vi "压力测试.vi"(15 "stop":bool) -> ()   [LabVIEW 2010]
uses:
  Instance           1 16Saved   压力测试 .vi
  Instance           2 16Saved   压力测试 .vi
  <vilib>/Analysis/NI_AALBase.lvlib
panel:
  in  "量  程(MPa)":dbl=5.0
  in  "零点输出(mV)":dbl=0.183
  in  "输出灵敏度（mV/V）":dbl=1.399
  out "当前压力值(MPa)":dbl(knob)=1.5270779105911612 scale=0.0..5.0
  out "压力 (Mpa)":dbl(graph)=1.31 caption="压力曲线 (Mpa)"
  # "压力测量实验"
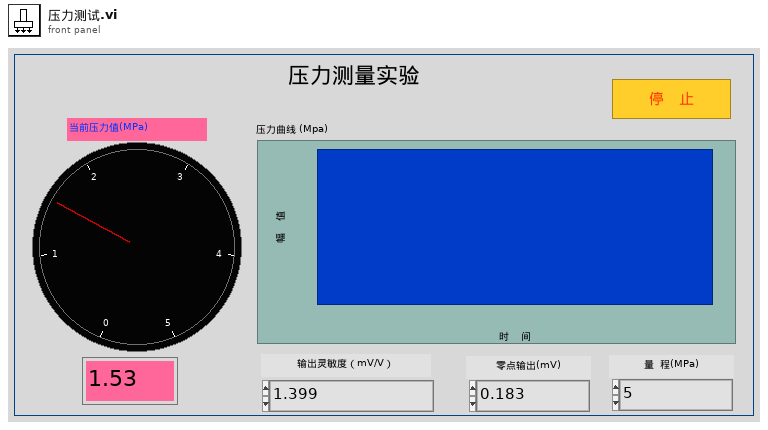
[diagram p1: front panel]
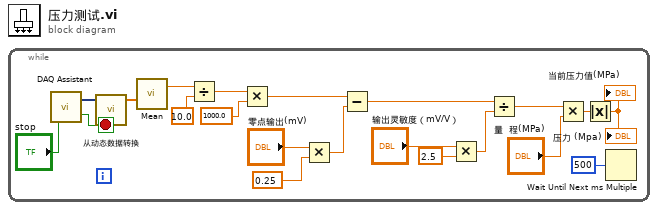
[diagram p0: block diagram]
diagram:
  n1 = while {
    stop <- w1 stop-if-true
    n2 = call "DAQ Assistant"("stop (F)"="stop") -> ("data"=w11:dynamicdata, "stopped"=w1:bool)  [unwired: 15 in, 2 out]
    n3 = call "从动态数据转换"("Dynamic Data Type"=w11) -> ("Array"=w10:dbl[])  [unwired: 3 in]
    n4 = call <vilib>:"Mean.vi"("X"=w10) -> ("mean"=w19:dbl)  [unwired: 1 out]
    n5 = Divide(x=w19, y=10.0) -> (x/y=w8:dbl)
    n6 = Multiply(x=w8, y=1000.0) -> (x*y=w18:dbl)
    n7 = Multiply(x="零点输出(mV)", y=0.25) -> (x*y=w16:dbl)
    n8 = Subtract(x=w18, y=w16) -> (x-y=w21:dbl)
    n9 = Multiply(x="输出灵敏度（mV/V）", y=2.5) -> (x*y=w14:dbl)
    n10 = Divide(x=w21, y=w14) -> (x/y=w20:dbl)
    n11 = Multiply(x=w20, y="量  程(MPa)") -> (x*y=w12:dbl)
    n12 = Absolute Value(x=w12) -> (abs(x)=→"压力 (Mpa)" →"当前压力值(MPa)":dbl)
    n13 = Wait Until Next ms Multiple(millisecond multiple=u32 500 ("毫秒倍数")) -> ()  [unwired: 1 out]
  }
